vi "User Info Message Callback.vi"(7 "Owner":refnum<class>, 11 "Message":refnum<class "Message.lvclass">) -> (0 "error out":errorcluster)   [LabVIEW 2020, in "LV Chat Client.lvclass"]
uses:
  LV Chat Client.lvclass
  <vilib>/IlluminatedG/lv-msg-simple/Stream-Simple-Msg/Message/Message.lvclass
  Data Types/User Info.ctl
  LV Chat Client.lvclass/LV Chat Client.ctl
  7c4e71ce-5648-4df2-8a80-a1e8a0151380.vi
  <vilib>/IlluminatedG/lv-msg-simple/Stream-Simple-Msg/Message/Data and Type.vi
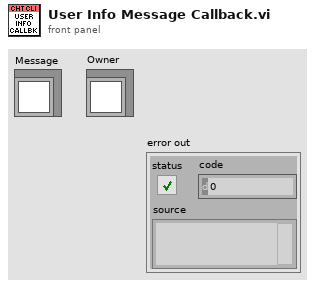
[diagram p1: front panel]
types:
  T1 = typedef "User Info.ctl" = cluster{"Name":string}
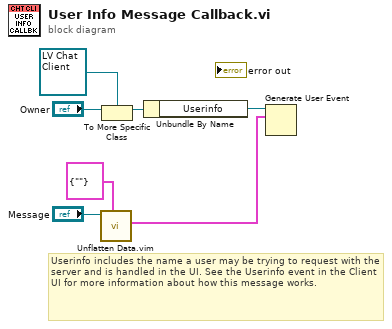
[diagram p0: block diagram]
diagram:
  # "Userinfo includes the name a user may be trying to request with the server and is handled in the UI. See the Userinfo event in the Client UI for more information about how this message works."
  n1 = call "Unflatten Data.vim"("Data Type (String)"=T1 {"Name"=""} ("User Info"), "Message in"="Message") -> ("Unflattened Data"=w1:T1)  [unwired: 7 in, 2 out]
  n2 = To More Specific Class(target class=refnum<class "LV Chat Client.lvclass"> refnum ("LV Chat Client.lvclass"), reference="Owner") -> (specific class reference=w4:refnum<class "LV Chat Client.lvclass">)  [unwired: 1 in, 1 out]
  n3 = Unbundle By Name(w4) -> ("Userinfo"=w2:refnum<user-event>)
  n4 = Generate User Event(user event=w2, event data cluster=w1) -> ()  [unwired: 2 in, 2 out]
